vi "TWEEZ MAIN.vi"() -> ()   [LabVIEW 2018]
uses:
  <vilib>/Utility/file.llb/Write Delimited Spreadsheet (I64).vi
panel:
  out "XYZsquared":cluster{i16, i16, i16}[](array[cluster])
  out "XYZ":cluster{i16, i16, i16}[](array[cluster])
  in  "Save":bool
  in  "Saving Path":path
  out "XYZ St. dev.":cluster{dbl, dbl, dbl}
  out "UDP Response":string
  out "FW Version":string
  in  "Reset Graph":bool
  out "Connected":bool
  in  "PI reset":bool
  in  "Enable PI":bool
  in  "PI parameters":T1
  in  "Parameter":string
  in  "WIPE":bool
  in  "CPAR":bool
  in  "Write custom command":bool
  in  "Custom Command":string
  in  "History Length":i32=20
  in  "stop":bool
  out "Bead Position":cluster{i16, i16}[](graph)
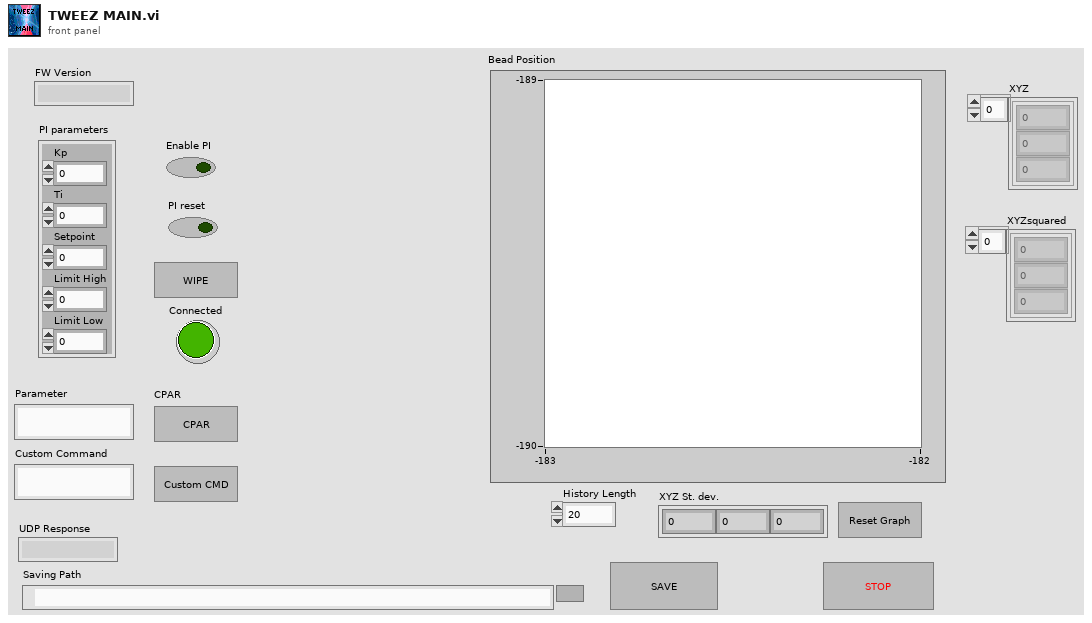
[diagram p1: front panel]
types:
  T1 = cluster{"Kp":dbl, "Ti":dbl, "Setpoint":dbl, "Limit High":dbl, "Limit Low":dbl}
  T2 = cluster{"name (unnamed)":string, "name (unnamed)":string}
  T3 = cluster{"name (unnamed)":string, "Variant":variant}
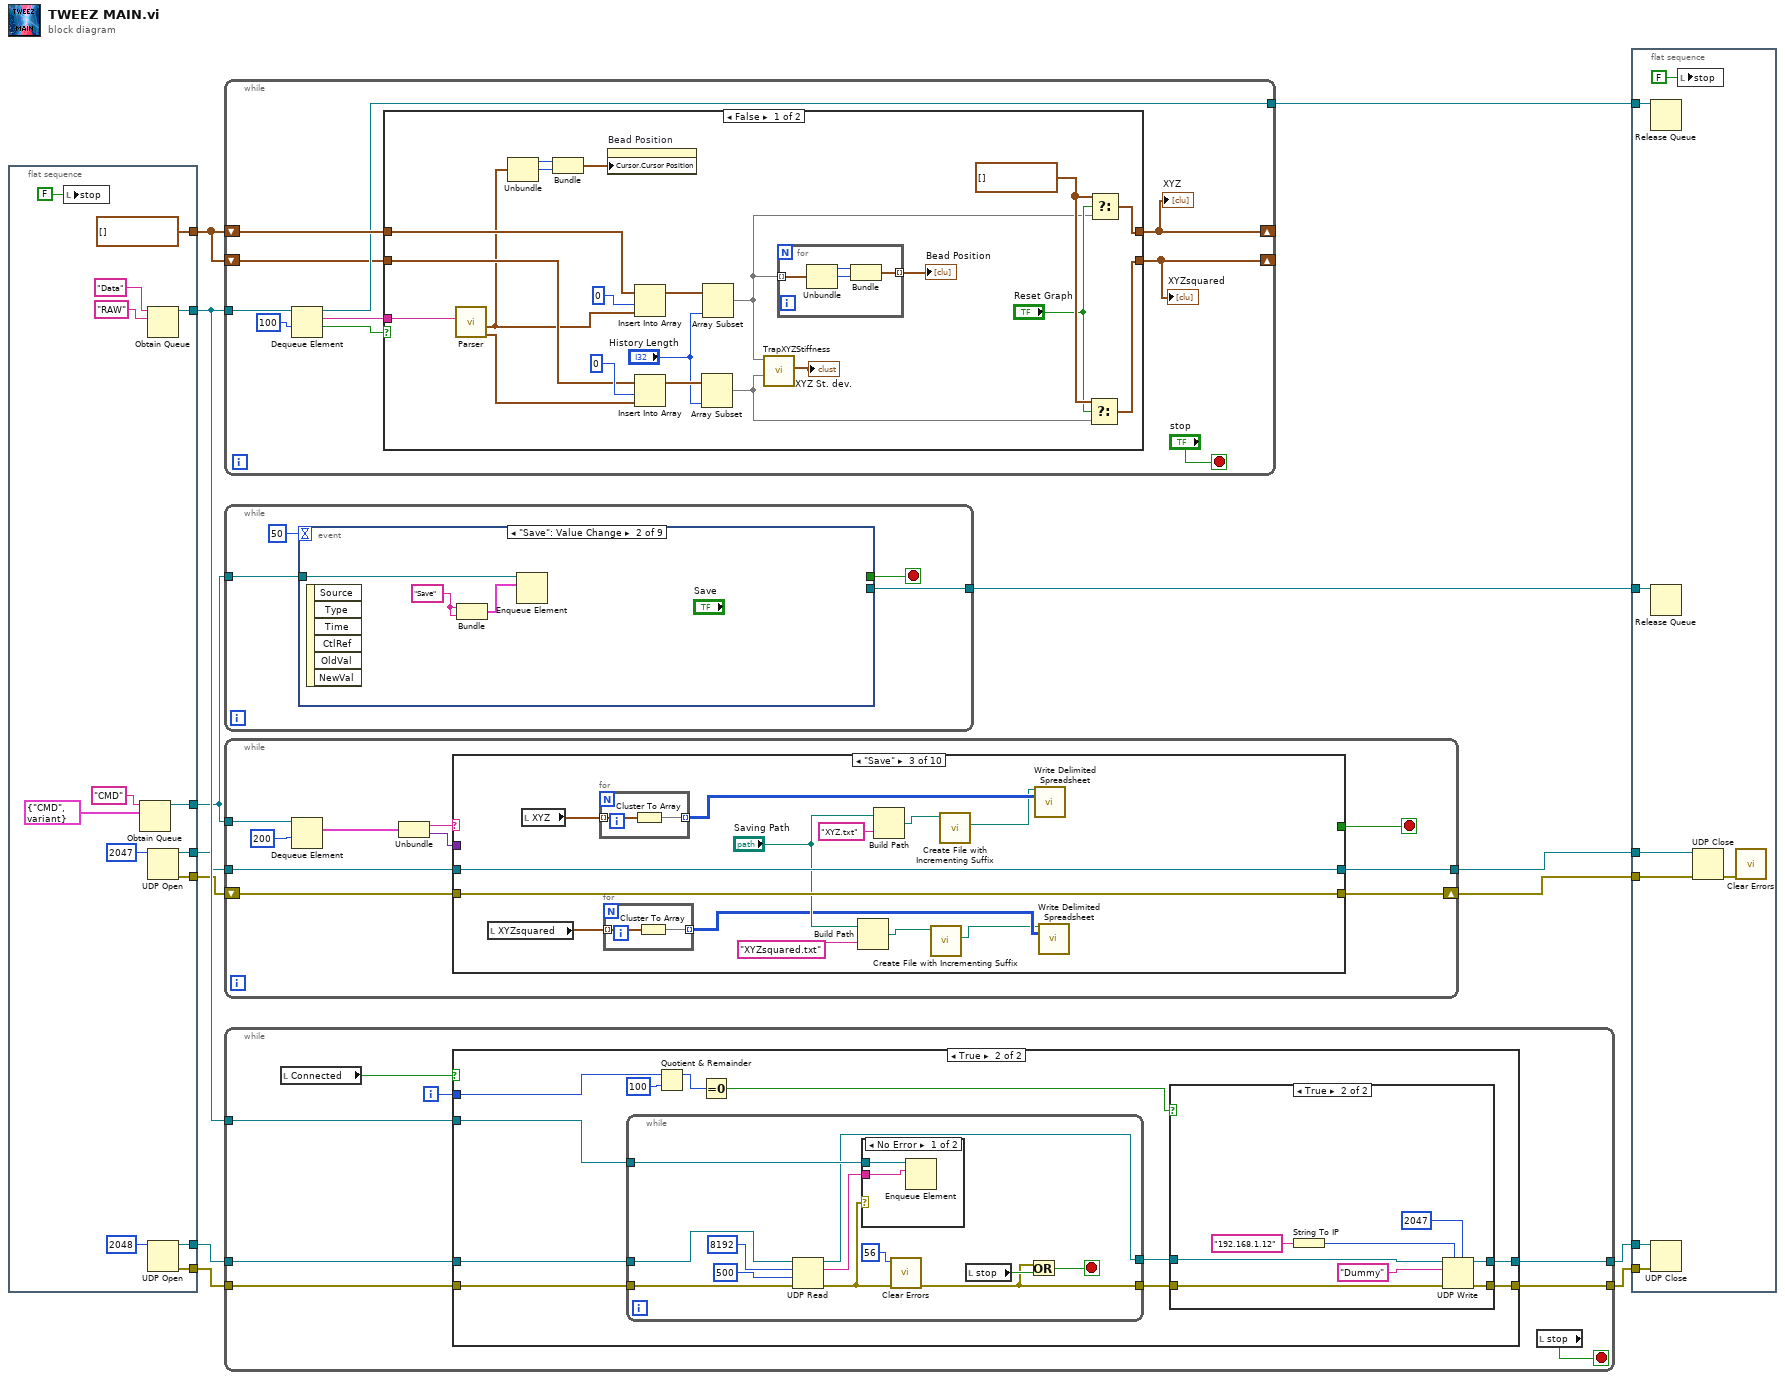
[diagram p0: block diagram]
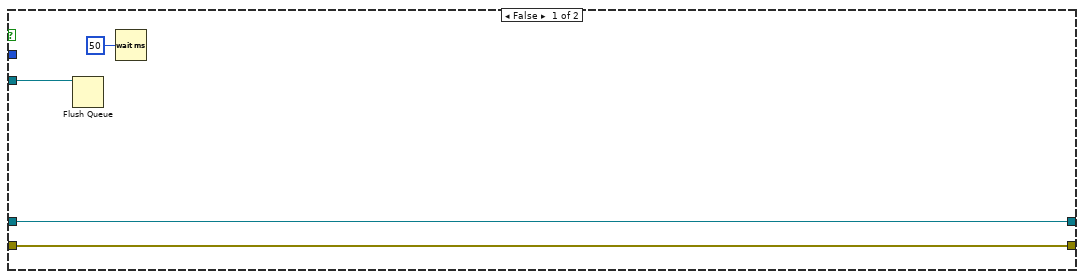
[diagram p2: hidden frame]
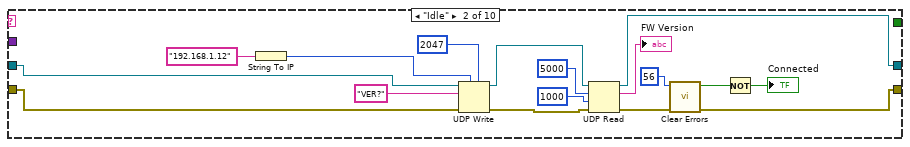
[diagram p6: hidden frame]
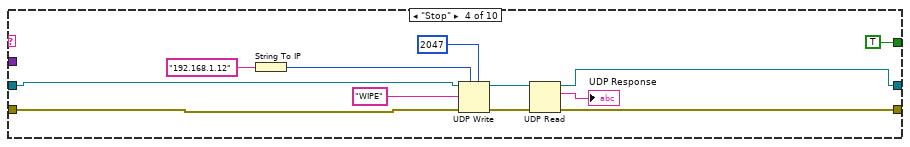
[diagram p7: hidden frame]
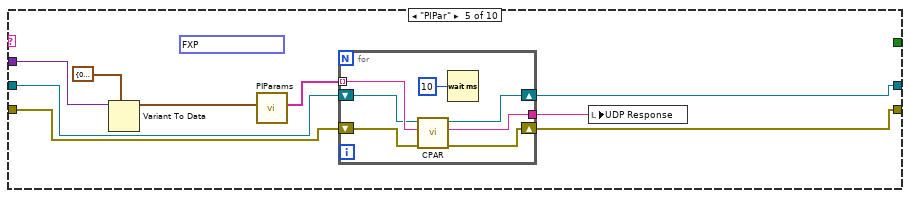
[diagram p8: hidden frame]
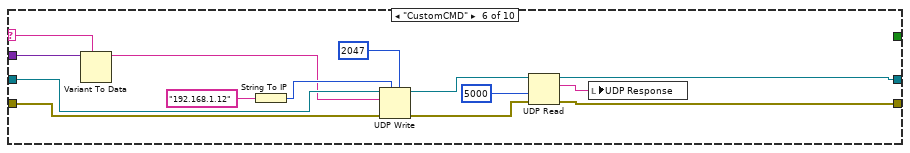
[diagram p9: hidden frame]
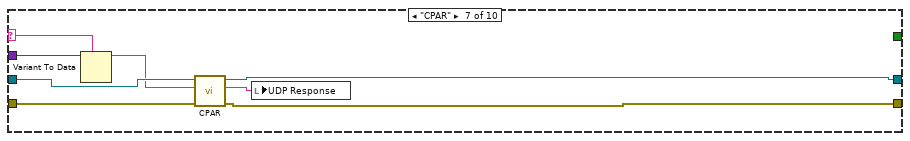
[diagram p10: hidden frame]
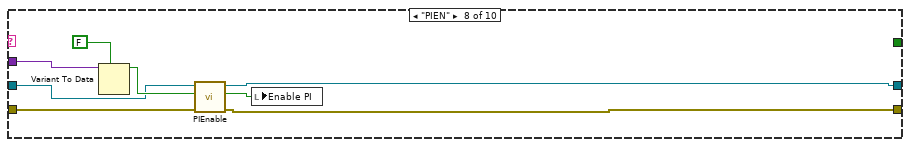
[diagram p11: hidden frame]
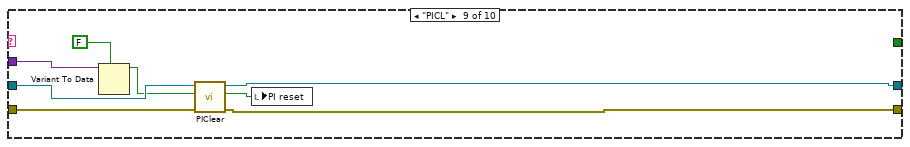
[diagram p12: hidden frame]
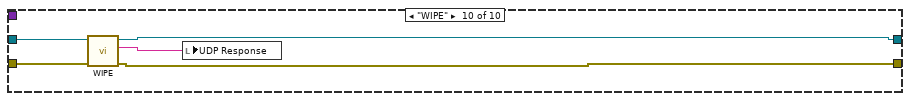
[diagram p13: hidden frame]
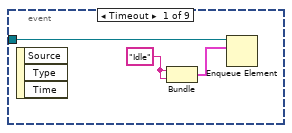
[diagram p14: hidden frame]
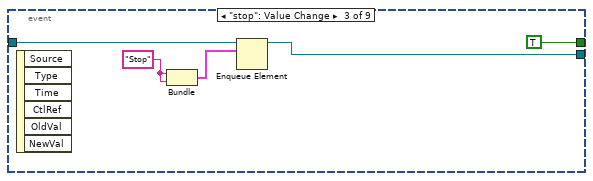
[diagram p15: hidden frame]
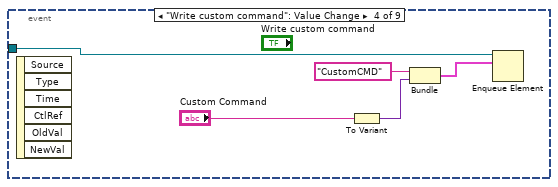
[diagram p16: hidden frame]
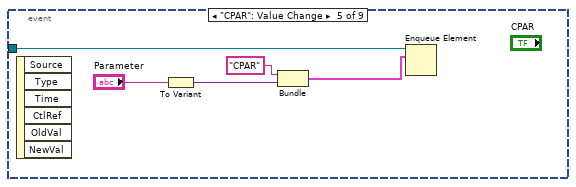
[diagram p17: hidden frame]
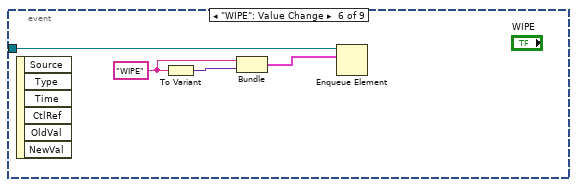
[diagram p18: hidden frame]
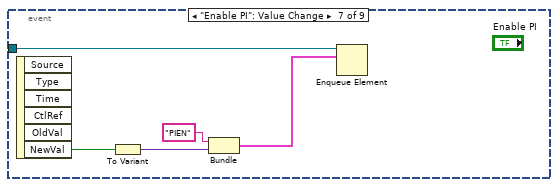
[diagram p19: hidden frame]
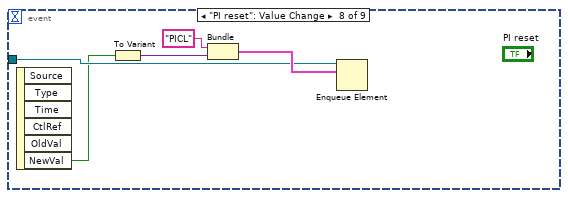
[diagram p20: hidden frame]
diagram:
  n1 = flat-sequence {
    tunnel: [w26] -> w6
    tunnel: [w25] -> w13
    tunnel: [w22] -> w12
    tunnel: [w18] -> w3
    tunnel: [w16] -> w11
    tunnel: [w15] -> w10
    tunnel: [cluster{i16, i16, i16}[] []] -> w1
    frame #0 {
      n2 = local write "stop"(FALSE ("stop")) -> ()
      n3 = Obtain Queue(name (unnamed)="CMD", element data type=cluster{"name (unnamed)":string, variant} {"name (unnamed)"="CMD", variant}) -> (queue out=w18:refnum<queue>)  [unwired: 3 in, 2 out]
      n4 = Obtain Queue(name (unnamed)="Data", element data type="RAW" ("name (unnamed)")) -> (queue out=w22:refnum<queue>)  [unwired: 3 in, 2 out]
      n5 = UDP Open(11:u16 2047 ("port")) -> (port=w16:refnum<k16>, 0:w15:errorcluster)  [unwired: 4 in, 1 out]
      n6 = UDP Open(11:u16 2048 ("port")) -> (port=w26:refnum<k16>, 0:w25:errorcluster)  [unwired: 4 in, 1 out]
    }
  }
  n7 = while {
    shift-right: [w35] -> _
    shift-left: w1 -> [w37]
    tunnel: w12 -> [w36]
    tunnel: [w31] -> w4
    shift-right: [w28] -> _
    shift-left: w1 -> [w29]
    stop <- "stop" stop-if-true
    n8 = Dequeue Element(queue=w36, timeout in ms (-1)=100) -> (queue out=w31:refnum<queue>, element=w30:string, timed out?=w33:bool)  [unwired: 1 in, 1 out]
    n9 = case shown="False" w33 {
      tunnel: w37 -> [w58 w64]
      tunnel: [w55 w64] -> w35
      tunnel: w30 -> [w54 _]
      tunnel: w29 -> [w52 w63]
      tunnel: [w46 w63] -> w28
      frame False {
        w50 = cluster{i16, i16, i16}[] []
        n10 = call "Parser.vi"("Raw data"=w54) -> ("XYZsquared"=w51:cluster{"X":i16, "Y":i16, "Z":i16}, "XYZ"=w43:cluster{"X":i16, "Y":i16, "Z":i16})  [unwired: 7 in, 2 out]
        n11 = Unbundle(w43) -> ("X"=w42:i16, "Y"=w41:i16)  [unwired: 1 out]
        n12 = Bundle("X"=w42, "Y"=w41) -> (w40:cluster{"X":i16, "Y":i16})  [unwired: 1 in]
        n13 = property on="Bead Position" class="XYGraph (strict)"("Cursor.Cursor Position"=w40) -> ()  [unwired: 2 in, 2 out]
        n14 = Insert Into Array(array=w58, index=0, new element=w43) -> (w57:cluster{i16, i16, i16}[])
        n15 = Insert Into Array(array=w52, index=0, new element=w51) -> (w48:cluster{i16, i16, i16}[])
        n16 = Array Subset(array=w48, length="History Length") -> (w45:cluster{i16, i16, i16}[])  [unwired: 1 in]
        n17 = Array Subset(array=w57, length="History Length") -> (w44:cluster{i16, i16, i16}[])  [unwired: 1 in]
        n18 = call "TrapXYZStiffness.vi"("XYZ Squared"=w45, "XYZ"=w44) -> ("XYZ St. dev."=→"XYZ St. dev.":cluster{dbl, dbl, dbl})  [unwired: 9 in]
        n19 = for {
          tunnel: w44 -> [w60] mode=indexing
          tunnel: [w59] -> w39 mode=indexing
          n20 = Unbundle(w60) -> (w61:i16, w62:i16)  [unwired: 1 out]
          n21 = Bundle(w61, w62) -> (w59:cluster{i16, i16})  [unwired: 1 in]
        }
        "Bead Position" <- w39
        n22 = Select(t=w50, s="Reset Graph", f=w45) -> (s? t:f=w46:cluster{i16, i16, i16}[])
        n23 = Select(t=w50, s="Reset Graph", f=w44) -> (s? t:f=w55:cluster{i16, i16, i16}[])
      }
      frame True {
        n24 = Wait (ms)(milliseconds to wait=u32 100) -> ()  [unwired: 1 out]
      }
    }
    "XYZ" <- w35
    "XYZsquared" <- w28
  }
  n25 = while {
    tunnel: w3 -> [w68]
    tunnel: [w66] -> w2
    stop <- w67 stop-if-true
    n26 = event shown="[1] \"Save\": Value Change" {
      selector: _ -> [_ _ _ _ _ _ _ _ _]
      dyn-events: _ -> [_ _ _ _ _ _ _ _ _]
      timeout: 50 ("milliseconds to wait") -> [_ _ _ _ _ _ _ _ _]
      tunnel: [_ _ TRUE _ _ _ _ _ _] -> w67
      tunnel: w68 -> [w71 w74 w77 w83 w88 w93 w96 w101 w109]
      tunnel: [_ _ w76 _ _ _ _ _ _] -> w66
      event Timeout {
        w70 = "Idle" ("name (unnamed)")
        n27 = event-data() -> ()  [unwired: 1 in, 3 out]
        n28 = Bundle("name (unnamed)"=w70, "name (unnamed)"=w70) -> (w72:T2)  [unwired: 1 in]
        n29 = Enqueue Element(queue=w71, element=w72) -> ()  [unwired: 2 in, 3 out]
      }
      event "Save": Value Change {
        w73 = "Save" ("name (unnamed)")
        n30 = event-data() -> ()  [unwired: 1 in, 6 out]
        n31 = Bundle("name (unnamed)"=w73, "name (unnamed)"=w73) -> (w75:T2)  [unwired: 1 in]
        n32 = Enqueue Element(queue=w74, element=w75) -> ()  [unwired: 2 in, 3 out]
      }
      event "stop": Value Change {
        w78 = "Stop" ("name (unnamed)")
        n33 = event-data() -> ()  [unwired: 1 in, 6 out]
        n34 = Bundle("name (unnamed)"=w78, "name (unnamed)"=w78) -> (w79:T2)  [unwired: 1 in]
        n35 = Enqueue Element(queue=w77, element=w79) -> (queue out=w76:refnum<queue>)  [unwired: 2 in, 2 out]
      }
      event "Write custom command": Value Change {
        n36 = event-data() -> ()  [unwired: 1 in, 6 out]
        n37 = To Variant(anything="Custom Command") -> (Variant=w81:variant)
        n38 = Bundle("name (unnamed)"="CustomCMD", "Variant"=w81) -> (w85:T3)  [unwired: 1 in]
        n39 = Enqueue Element(queue=w83, element=w85) -> ()  [unwired: 2 in, 3 out]
      }
      event "CPAR": Value Change {
        n40 = event-data() -> ()  [unwired: 1 in, 6 out]
        n41 = To Variant(anything="Parameter") -> (Variant=w87:variant)
        n42 = Bundle("name (unnamed)"="CPAR", "Variant"=w87) -> (w90:T3)  [unwired: 1 in]
        n43 = Enqueue Element(queue=w88, element=w90) -> ()  [unwired: 2 in, 3 out]
      }
      event "WIPE": Value Change {
        w91 = "WIPE" ("name (unnamed)")
        n44 = event-data() -> ()  [unwired: 1 in, 6 out]
        n45 = To Variant(anything=w91) -> (Variant=w92:variant)
        n46 = Bundle("name (unnamed)"=w91, "Variant"=w92) -> (w94:T3)  [unwired: 1 in]
        n47 = Enqueue Element(queue=w93, element=w94) -> ()  [unwired: 2 in, 3 out]
      }
      event "Enable PI": Value Change {
        n48 = event-data() -> ("NewVal"=w95:bool)  [unwired: 1 in, 5 out]
        n49 = To Variant(anything=w95) -> (Variant=w98:variant)
        n50 = Bundle("name (unnamed)"="PIEN", "Variant"=w98) -> (w99:T3)  [unwired: 1 in]
        n51 = Enqueue Element(queue=w96, element=w99) -> ()  [unwired: 2 in, 3 out]
      }
      event "PI reset": Value Change {
        n52 = event-data() -> ("NewVal"=w100:bool)  [unwired: 1 in, 5 out]
        n53 = To Variant(anything=w100) -> (Variant=w103:variant)
        n54 = Bundle("name (unnamed)"="PICL", "Variant"=w103) -> (w104:T3)  [unwired: 1 in]
        n55 = Enqueue Element(queue=w101, element=w104) -> ()  [unwired: 2 in, 3 out]
      }
      event "PI parameters": Value Change {
        n56 = event-data() -> ("NewVal"=w107:T1)  [unwired: 1 in, 5 out]
        n57 = To Variant(anything=w107) -> (Variant=w106:variant)
        n58 = Bundle("name (unnamed)"="PIPar", "Variant"=w106) -> (w108:T3)  [unwired: 1 in]
        n59 = Enqueue Element(queue=w109, element=w108) -> ()  [unwired: 2 in, 3 out]
      }
    }
  }
  n60 = while {
    tunnel: w3 -> [w119]
    tunnel: w11 -> [w114]
    shift-right: [w112] -> w8
    shift-left: w10 -> [w113]
    tunnel: [w111] -> w9
    stop <- w116 stop-if-true
    n61 = Dequeue Element(queue=w119, timeout in ms (-1)=200) -> (element=w118:cluster{"name (unnamed)":string, variant})  [unwired: 1 in, 3 out]
    n62 = Unbundle(w118) -> ("name (unnamed)"=w117:string, w110:variant)
    n63 = case shown="\"Save\"" w117 {
      selector: w117 -> [_ _ _ _ _ w196 w204 _ _ _]
      tunnel: [_ _ _ TRUE _ _ _ _ _ _] -> w116
      tunnel: w114 -> [w121 w134 w151 w162 w172 w192 w203 w210 w219 w226]
      tunnel: w113 -> [w120 w133 w150 w161 w171 w190 w201 w209 w217 w224]
      tunnel: [w120 w130 w150 w157 w169 w186 w200 w208 w216 w223] -> w112
      tunnel: [w121 w127 w151 w158 w170 w185 w199 w207 w215 w225] -> w111
      tunnel: w110 -> [_ _ _ _ w176 w197 w205 w213 w221 _]
      frame "unknown", Default {
      }
      frame "Idle" {
        n64 = String To IP(1:"192.168.1.12" ("name")) -> (0:w137:u32)
        n65 = UDP Write(address=w137, port or service name=u16 2047, connection ID=w134, data in="VER?", 8:w133) -> (error out=w126:errorcluster, 3:w129:refnum<k16>)  [unwired: 1 in]
        n66 = UDP Read(connection ID=w129, max size (548)=5000 ("timeout ms (25000)"), timeout ms (25000)=1000, 8:w126) -> (data out=→"FW Version":string, error out=w128:errorcluster, 3:w127:refnum<k16>)  [unwired: 2 out]
        n67 = call <vilib>:"Clear Errors.vi"("error in (no error)"=w128, "specific error code to clear (0: all)"=56) -> ("error out"=w130:errorcluster, "specific error cleared?"=w132:bool)  [unwired: 4 in]
        n68 = Not(x=w132) -> (.not. x?=→"Connected":bool)
      }
      frame "Save" {
        n69 = local read "XYZsquared"() -> (w149:cluster{i16, i16, i16}[])
        n70 = local read "XYZ"() -> (w139:cluster{i16, i16, i16}[])
        n71 = for {
          tunnel: w139 -> [w155] mode=indexing
          tunnel: [w154] -> w148 mode=indexing
          n72 = Cluster To Array(cluster=w155) -> (array=w154:i16[])
        }
        n73 = for {
          tunnel: w149 -> [w153] mode=indexing
          tunnel: [w152] -> w145 mode=indexing
          n74 = Cluster To Array(cluster=w153) -> (array=w152:i16[])
        }
        n75 = Build Path(base path="Saving Path", name or relative path="XYZsquared.txt") -> (appended path=w141:path)
        n76 = Build Path(base path="Saving Path", name or relative path="XYZ.txt") -> (appended path=w143:path)
        n77 = call <vilib>:"Create File with Incrementing Suffix.vi"("file path"=w141) -> ("actual path"=w140:path)  [unwired: 8 in, 2 out]
        n78 = call <vilib>:"Create File with Incrementing Suffix.vi"("file path"=w143) -> ("actual path"=w142:path)  [unwired: 8 in, 2 out]
        n79 = call-poly <vilib>:"Write Delimited Spreadsheet.vi"("file path (dialog if empty)"=w142, "2D data"=w148) -> ()  [unwired: 12 in, 2 out]
        n80 = call-poly <vilib>:"Write Delimited Spreadsheet.vi"("file path (dialog if empty)"=w140, "2D data"=w145) -> ()  [unwired: 12 in, 2 out]
      }
      frame "Stop" {
        n81 = String To IP(1:"192.168.1.12" ("name")) -> (0:w165:u32)
        n82 = UDP Write(address=w165, port or service name=u16 2047, connection ID=w162, data in="WIPE", 8:w161) -> (error out=w159:errorcluster, 3:w160:refnum<k16>)  [unwired: 1 in]
        n83 = UDP Read(connection ID=w160, 8:w159) -> (data out=→"UDP Response":string, error out=w157:errorcluster, 3:w158:refnum<k16>)  [unwired: 2 in, 2 out]
      }
      frame "PIPar" {
        (unwired) fxp<+/-,16,1> 0.160003662109375 ("fixed-point type")
        n84 = Variant To Data(type=T1 {"Kp"=0.0, "Ti"=0.0, "Setpoint"=0.0, "Limit High"=0.0, "Limit Low"=0.0} ("PI parameters"), Variant=w176) -> (data=w174:T1)  [unwired: 1 in, 1 out]
        n85 = call "PIParams.vi"("PI parameters"=w174) -> ("Params Out"=w173:string[])  [unwired: 10 in]
        n86 = for {
          tunnel: w173 -> [w183] mode=indexing
          shift-right: [w179] -> w169
          shift-left: w171 -> [w181]
          shift-right: [w180] -> w170
          shift-left: w172 -> [w182]
          tunnel: [w177] -> w168
          n87 = call "CPAR.vi"("error in (no error)"=w181, "Parameter"=w183, "connection ID"=w182) -> ("error out"=w179:errorcluster, "data out"=w177:string, "connection ID out"=w180:refnum<k16>)  [unwired: 6 in]
          n88 = Wait (ms)(milliseconds to wait=u32 10) -> ()  [unwired: 1 out]
        }
        n89 = local write "UDP Response"(w168) -> ()
      }
      frame "CustomCMD" {
        n90 = Variant To Data(type=w196, Variant=w197) -> (data=w191:string)  [unwired: 1 in, 1 out]
        n91 = String To IP(1:"192.168.1.12" ("name")) -> (0:w195:u32)
        n92 = UDP Write(address=w195, port or service name=u16 2047, connection ID=w192, data in=w191, 8:w190) -> (error out=w187:errorcluster, 3:w188:refnum<k16>)  [unwired: 1 in]
        n93 = UDP Read(connection ID=w188, timeout ms (25000)=5000, 8:w187) -> (data out=w184:string, error out=w186:errorcluster, 3:w185:refnum<k16>)  [unwired: 1 in, 2 out]
        n94 = local write "UDP Response"(w184) -> ()
      }
      frame "CPAR" {
        n95 = Variant To Data(type=w204, Variant=w205) -> (data=w202:string)  [unwired: 1 in, 1 out]
        n96 = call "CPAR.vi"("error in (no error)"=w201, "Parameter"=w202, "connection ID"=w203) -> ("error out"=w200:errorcluster, "data out"=w198:string, "connection ID out"=w199:refnum<k16>)  [unwired: 6 in]
        n97 = local write "UDP Response"(w198) -> ()
      }
      frame "PIEN" {
        n98 = Variant To Data(type=FALSE ("stop"), Variant=w213) -> (data=w211:bool)  [unwired: 1 in, 1 out]
        n99 = call "PIEnable.vi"("error in (no error)"=w209, "Enable?"=w211, "connection ID"=w210) -> ("error out"=w208:errorcluster, "Enable"=w206:bool, "connection ID out"=w207:refnum<k16>)  [unwired: 6 in]
        n100 = local write "Enable PI"(w206) -> ()
      }
      frame "PICL" {
        n101 = Variant To Data(type=FALSE ("stop"), Variant=w221) -> (data=w218:bool)  [unwired: 1 in, 1 out]
        n102 = call "PIClear.vi"("error in (no error)"=w217, "Clear?"=w218, "connection ID"=w219) -> ("error out"=w216:errorcluster, "Clear"=w214:bool, "connection ID out"=w215:refnum<k16>)  [unwired: 6 in]
        n103 = local write "PI reset"(w214) -> ()
      }
      frame "WIPE" {
        n104 = call "WIPE.vi"("error in (no error)"=w224, "connection ID"=w226) -> ("error out"=w223:errorcluster, "data out"=w222:string, "connection ID out"=w225:refnum<k16>)  [unwired: 7 in]
        n105 = local write "UDP Response"(w222) -> ()
      }
    }
  }
  n106 = while {
    tunnel: w6 -> [w233]
    tunnel: w13 -> [w232]
    tunnel: w12 -> [w234]
    tunnel: [w229] -> w5
    tunnel: [w228] -> w7
    i -> [w227]
    stop <- w230 stop-if-true
    n107 = local read "Connected"() -> (w231:bool)
    n108 = case shown="True" w231 {
      tunnel: w234 -> [w235 w249]
      tunnel: w233 -> [w237 w248]
      tunnel: w232 -> [w236 w247]
      tunnel: [w237 w239] -> w229
      tunnel: [w236 w240] -> w228
      tunnel: w227 -> [_ w246]
      frame False {
        n109 = Flush Queue(queue=w235) -> ()  [unwired: 1 in, 3 out]
        n110 = Wait (ms)(milliseconds to wait=u32 50) -> ()  [unwired: 1 out]
      }
      frame True {
        n111 = while {
          tunnel: w249 -> [w271]
          tunnel: w248 -> [w269]
          tunnel: w247 -> [w268]
          tunnel: [w261] -> w242
          tunnel: [w260] -> w241
          stop <- w262 stop-if-true
          n112 = UDP Read(connection ID=w269, max size (548)=8192 ("timeout ms (25000)"), timeout ms (25000)=500, 8:w268) -> (data out=w266:string, error out=w264:errorcluster, 3:w261:refnum<k16>)  [unwired: 2 out]
          n113 = case shown="No Error" w264 {
            tunnel: w271 -> [w273 _]
            tunnel: w266 -> [w272 _]
            frame No Error {
              n114 = Enqueue Element(queue=w273, element=w272) -> ()  [unwired: 2 in, 3 out]
            }
            frame Error {
            }
          }
          n115 = call <vilib>:"Clear Errors.vi"("error in (no error)"=w264, "specific error code to clear (0: all)"=56) -> ("error out"=w260:errorcluster)  [unwired: 4 in, 1 out]
          n116 = local read "stop"() -> (w263:bool)
          n117 = Or(x=w260, y=w263) -> (x .or. y?=w262:bool)
        }
        n118 = Quotient & Remainder(x=w246, y=100) -> (x-y*floor(x/y)=w244:i32)  [unwired: 1 out]
        n119 = Equal To 0?(x=w244) -> (x = 0?=w243:bool)
        n120 = case shown="True" w243 {
          tunnel: w242 -> [w251 w259]
          tunnel: w241 -> [w250 w258]
          tunnel: [w250 w257] -> w240
          tunnel: [w251 w256] -> w239
          frame False {
          }
          frame True {
            n121 = String To IP(1:"192.168.1.12" ("name")) -> (0:w253:u32)
            n122 = UDP Write(address=w253, port or service name=u16 2047, connection ID=w259, data in="Dummy", 8:w258) -> (error out=w257:errorcluster, 3:w256:refnum<k16>)  [unwired: 1 in]
          }
        }
      }
    }
    n123 = local read "stop"() -> (w230:bool)
  }
  n124 = flat-sequence {
    tunnel: w5 -> [w280]
    tunnel: w7 -> [w281]
    tunnel: w2 -> [w279]
    tunnel: w9 -> [w276]
    tunnel: w8 -> [w275]
    tunnel: w4 -> [w277]
    frame #0 {
      n125 = Release Queue(queue=w277) -> ()  [unwired: 2 in, 3 out]
      n126 = Release Queue(queue=w279) -> ()  [unwired: 2 in, 3 out]
      n127 = UDP Close(connection ID=w280, 8:w281) -> ()  [unwired: 2 out]
      n128 = local write "stop"(FALSE ("stop")) -> ()
      n129 = UDP Close(connection ID=w276, 8:w275) -> (error out=w274:errorcluster)  [unwired: 1 out]
      n130 = call <vilib>:"Clear Errors.vi"("error in (no error)"=w274) -> ()  [unwired: 5 in, 2 out]
    }
  }
